vi "Hitrap_DiagnosticBox.Wait.vi"(0 "i ref in":refnum<vi>, 2 "Timeout":i32, 3 "Axis":i32, 5 "error in":errorcluster) -> (14 "i ref out":refnum<vi>, 17 "Timeout?":bool, 19 "error out":errorcluster)   [LabVIEW 2014, in "Hitrap_DiagnosticBox.lvlib"]
doc: "Wait until reference move stopped or the time out over.\n\nThis VI is used in \"GoToPosition\""
uses:
  Hitrap_DiagnosticBox.lvlib
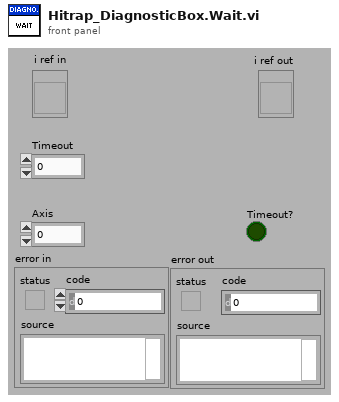
[diagram p1: front panel]
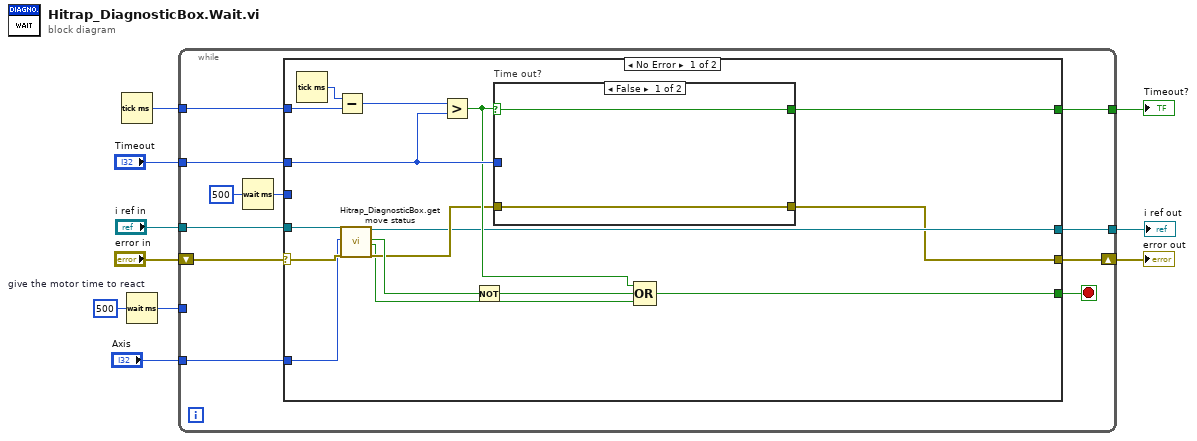
[diagram p0: block diagram]
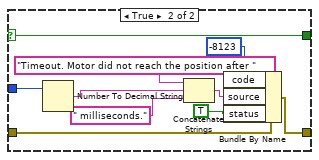
[diagram p2: hidden frame]
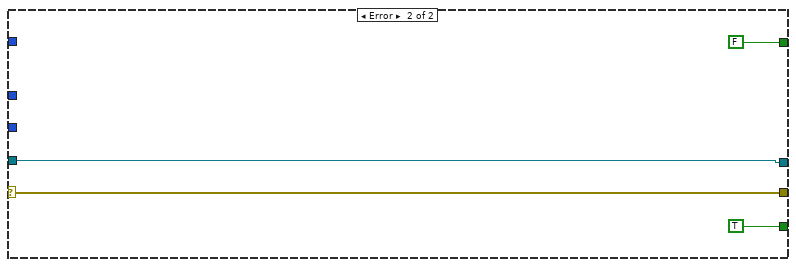
[diagram p3: hidden frame]
diagram:
  n1 = Tick Count (ms)() -> (millisecond timer value=w5:u32)
  n2 = Wait (ms) "give the motor time to react"(milliseconds to wait=u32 500) -> (millisecond timer value=w7:u32)
  n3 = while {
    shift-right: [w21] -> w10
    shift-left: "error in" -> [w19]
    tunnel: w7 -> [_]
    tunnel: "Timeout" -> [w18]
    tunnel: w5 -> [w17]
    tunnel: [w16] -> w4
    tunnel: "i ref in" -> [w15]
    tunnel: [w14] -> w2
    tunnel: "Axis" -> [w11]
    stop <- w20 stop-if-true
    n4 = Wait (ms)(milliseconds to wait=u32 500) -> (millisecond timer value=w12:u32)
    n5 = case shown="No Error" w19 {
      selector: w19 -> [w28 w53]
      tunnel: [w24 w53] -> w21
      tunnel: [w30 TRUE] -> w20
      tunnel: w18 -> [w33 _]
      tunnel: w17 -> [w36 _]
      tunnel: [w34 FALSE] -> w16
      tunnel: w15 -> [w29 w50]
      tunnel: [w25 w50] -> w14
      tunnel: w12 -> [_ _]
      tunnel: w11 -> [w22 _]
      frame No Error {
        n6 = Tick Count (ms)() -> (millisecond timer value=w37:u32)
        n7 = Subtract(x=w37, y=w36) -> (x-y=w35:u32)
        n8 = call "Hitrap_DiagnosticBox.get move status.vi"("i ref in"=w29, "Axis"=w22, "error in (no error)"=w28) -> ("i ref out"=w25:refnum<vi>, "Moving"=w27:bool, "Error"=w23:bool, "error out"=w26:errorcluster)  [unwired: 13 in]
        n9 = Greater?(x=w35, y=w33) -> (0:w31:bool)
        n10 = Not(x=w27) -> (.not. x?=w32:bool)
        n11 = case "Time out?" shown="False" w31 {
          selector: w31 -> [w38 w47]
          tunnel: [w39 w48] -> w24
          tunnel: [w38 w47] -> w34
          tunnel: w33 -> [_ w46]
          tunnel: w26 -> [w39 w41]
          frame False {
          }
          frame True {
            n12 = Number To Decimal String(number=w46) -> (decimal integer string=w44:string)  [unwired: 1 in]
            n13 = Concatenate Strings("Timeout. Motor did not reach the position after " ("source"), w44, " milliseconds." ("source")) -> (w42:string)
            n14 = Bundle By Name(cluster=w41, "code"=-8123, "source"=w42, "status"=TRUE) -> (w48:errorcluster)
          }
        }
        n15 = Compound Arithmetic op=OR(w31, w32, w23) -> (w30:bool)
      }
      frame Error {
      }
    }
  }
  "error out" <- w10
  "Timeout?" <- w4
  "i ref out" <- w2
